vi "buildMFCerrorMessage.vi"(9 "Mdot":dbl, 10 "OverallMinMdot(g/min)":dbl, 11 "OverallMaxMdot(g/min)":dbl) -> (3 "errorMessage":string)   [LabVIEW 2016]
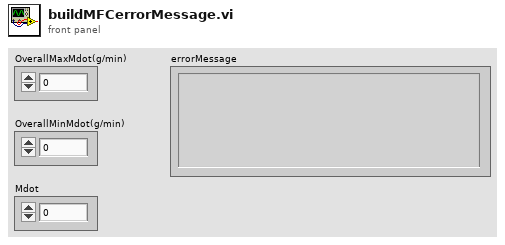
[diagram p1: front panel]
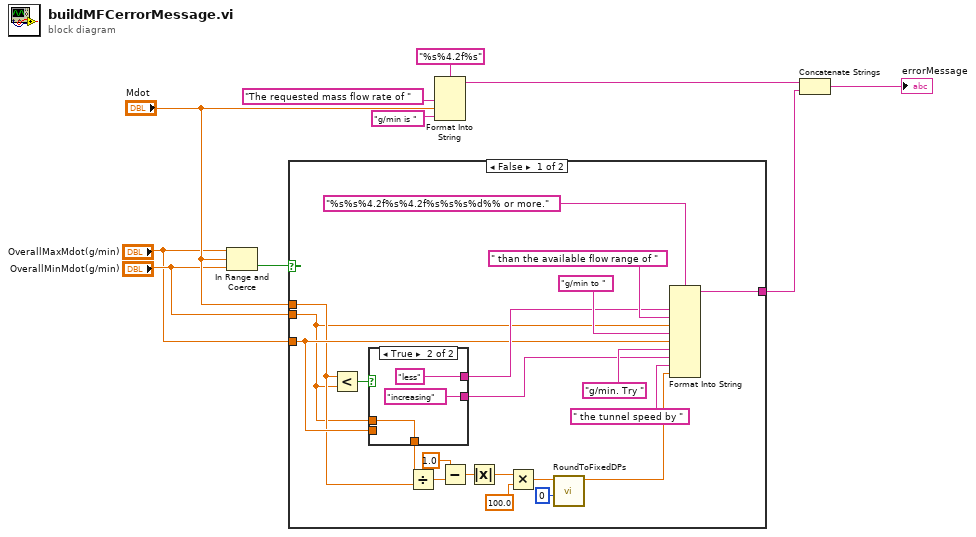
[diagram p0: block diagram]
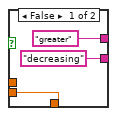
[diagram p2: hidden frame]
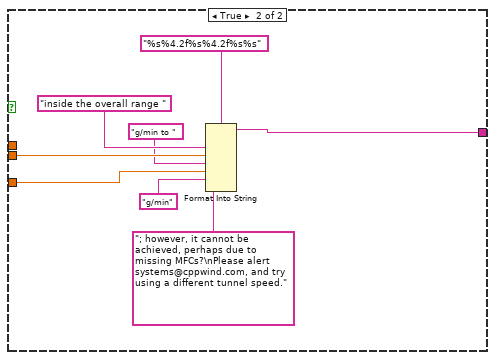
[diagram p3: hidden frame]
diagram:
  n1 = In Range and Coerce(upper limit="OverallMaxMdot(g/min)", x="Mdot", lower limit="OverallMinMdot(g/min)") -> (In Range?=w6:bool)  [unwired: 1 out]
  n2 = case shown="False" w6 {
    tunnel: "Mdot" -> [w14 _]
    tunnel: "OverallMinMdot(g/min)" -> [w13 w44]
    tunnel: "OverallMaxMdot(g/min)" -> [w22 w43]
    tunnel: [w27 w40] -> w1
    frame False {
      n3 = Less?(x=w14, y=w13) -> (x < y?=w26:bool)
      n4 = case shown="True" w26 {
        tunnel: ["greater" "less"] -> w25
        tunnel: ["decreasing" "increasing"] -> w24
        tunnel: w22 -> [w32 _]
        tunnel: [w32 w35] -> w15
        tunnel: w13 -> [_ w35]
        frame False {
        }
        frame True {
        }
      }
      n5 = Divide(x=w15, y=w14) -> (x/y=w17:dbl)
      n6 = Subtract(x=1.0, y=w17) -> (x-y=w16:dbl)
      n7 = Absolute Value(x=w16) -> (abs(x)=w12:dbl)
      n8 = Multiply(x=w12, y=100.0) -> (x*y=w20:dbl)
      n9 = call "RoundToFixedDPs.vi"("Power of ten"=0, "Number to round"=w20) -> ("Rounded number"=w11:dbl)  [unwired: 8 in, 1 out]
      n10 = Format Into String(format string="%s%s%4.2f%s%4.2f%s%s%s%d%% or more.", w25, " than the available flow range of ", w13, "g/min to " ("input 4"), w22, "g/min. Try " ("input 4"), w24, " the tunnel speed by ", w11) -> (resulting string=w27:string)  [unwired: 2 in, 1 out]
    }
    frame True {
      n11 = Format Into String(format string="%s%4.2f%s%4.2f%s%s", "inside the overall range ", w44, "g/min to " ("input 4"), w43, "g/min" ("input 4"), "; however, it cannot be achieved, perhaps due to missing MFCs?\nPlease alert systems@cppwind.com, and try using a different tunnel speed.") -> (resulting string=w40:string)  [unwired: 2 in, 1 out]
    }
  }
  n12 = Format Into String(format string="%s%4.2f%s", "The requested mass flow rate of ", "Mdot", "g/min is ") -> (resulting string=w7:string)  [unwired: 2 in, 1 out]
  n13 = Concatenate Strings(w7, w1) -> (→"errorMessage":string)
